vi "GraphsUpdateMeta.vi"(0 "raw graph ref":refnum<vi>, 1 "File Paths":T2={"Local Save Path"=path "\\\\smbhome.uscs.susx.ac.uk\\cv222/Desktop/data", "Newton Save Path"=path "Z:/#Projects/Entanglement/data", "File Name"="test", "LocalSave"=TRUE}, 3 "Compiler Settings":T1={"Python Path"=path "", "Main File"="mainscript.py", "Meta File"="metascript.txt", "Aux File"="auxscript.py", "Pre File"="metascript.txt"}, 5 "mean graph ref":refnum<vi>, 7 "proc graph ref":refnum<vi>, 11 "error in (no error)":errorcluster, 12 "ControllerSettingsRef":refnum<vi>) -> (15 "error out":errorcluster)   [LabVIEW 2019]
uses:
  controls/FilePaths.ctl
  PulseCompiler/CompilerSettings.ctl
  controls/ControllerSettings.ctl
  controls/GlobalExp.vi
  Global.lvlib
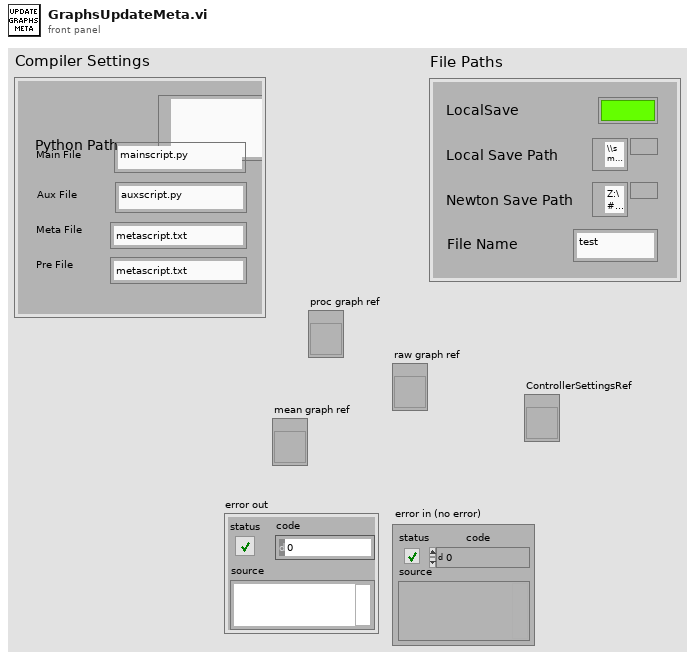
[diagram p1: front panel]
types:
  T1 = typedef "CompilerSettings.ctl" = cluster{"Python Path":path, "Main File":string, "Meta File":string, "Aux File":string, "Pre File":string}
  T2 = typedef "FilePaths.ctl" = cluster{"Local Save Path":path, "Newton Save Path":path, "File Name":string, "LocalSave":bool}
  T3 = typedef "MasterExpControl.ctl" = cluster{"Main Steps":dbl, "Main Runs":dbl, "ExpStatus":enum16{"Innit", "Stop", "Idle", "MainRunning", "AuxRunning"}, "Main Current Step":dbl, "ExpNum":dbl, "NewData":bool, "date":string, "command":string, "Stop":bool, "Pause":bool, "Mathematica":string, "Main/Meta":bool, "UpdateMath":bool, "Camera":bool, "MetaExpOver":bool, "NextMetaExp":bool}
  T4 = typedef "ControllerSettings.ctl" = cluster{"Aux Sequence":bool, "Camera":bool, "Recrystallize":bool, "Raw graph":bool, "Mean graph":bool, "Calculate probs":bool, "Find fit":bool, "ReX Time [s] :":dbl, "Lock Voltage :":dbl, "Line trig ":bool, "Check Fluo":bool, "Pre Sequence":bool}
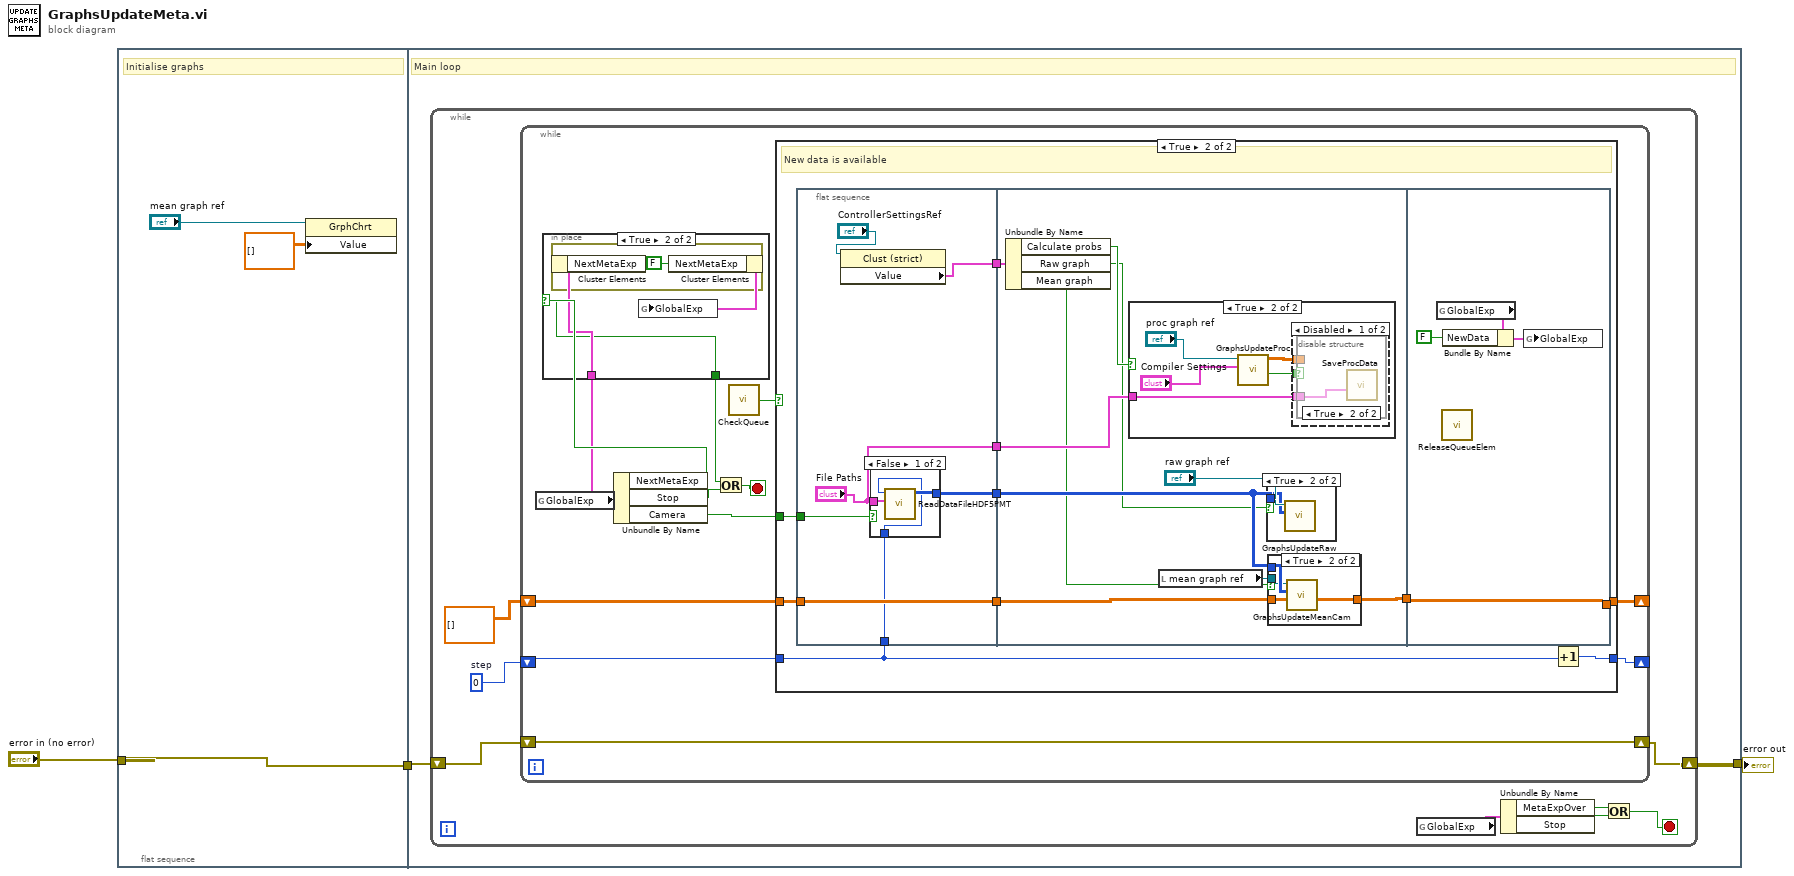
[diagram p0: block diagram]
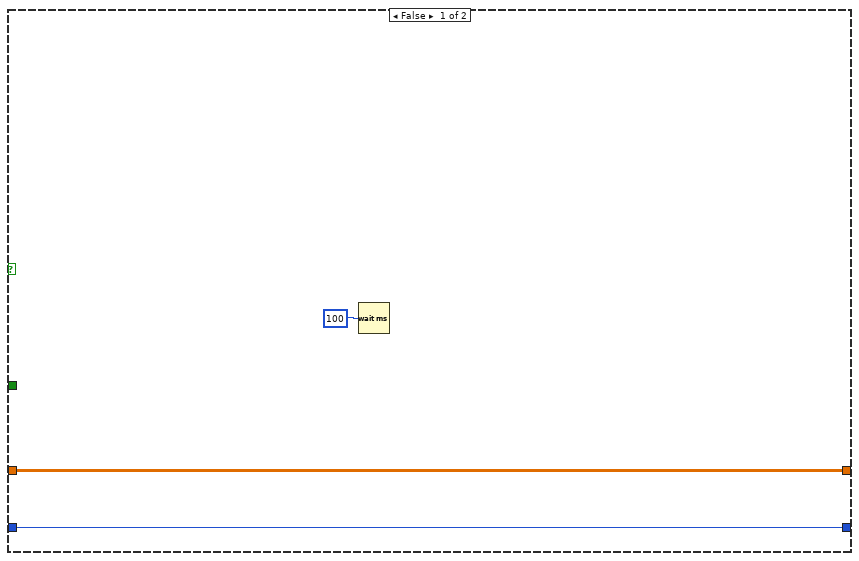
[diagram p3: hidden frame]
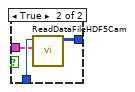
[diagram p4: hidden frame]
diagram:
  n1 = flat-sequence {
    tunnel: "error in (no error)" -> [w6]
    tunnel: [w6] -> w1
    tunnel: [w7] -> w2
    tunnel: w1 -> [w8]
    frame #0 {
      # "Initialise graphs"
      n2 = property class="GrphChrt"(reference="mean graph ref", "Value"=dbl[][] []) -> ()  [unwired: 1 in, 2 out]
    }
    frame #1 {
      # "Main loop"
      n3 = while {
        shift-right: [w15] -> w7
        shift-left: w8 -> [w16]
        stop <- w9 stop-if-true
        w14 = 0  # step
        n4 = while {
          shift-right: [w28] -> w15
          shift-left: w16 -> [w28]
          shift-right: [w24] -> _
          shift-left: w14 -> [w25]
          shift-right: [w22] -> _
          shift-left: dbl[][] [] -> [w23]
          stop <- w17 stop-if-true
          n5 = global read "GlobalExp.vi" "GlobalExp"() -> (w20:T3)
          n6 = Unbundle By Name(w20) -> ("NextMetaExp"=w21:bool, "Stop"=w18:bool, "Camera"=w27:bool)
          n7 = case shown="True" w21 {
            selector: w21 -> [w29 w30]
            tunnel: w20 -> [_ w32]
            tunnel: [w29 w30] -> w19
            frame False {
            }
            frame True {
              n8 = in-place {
                n9 = in-place-cluster #1(w32) -> ()  [unwired: 1 out]
                n10 = in-place-cluster #1("NextMetaExp"=FALSE) -> (w31:T3)
              }
              n11 = global write "GlobalExp.vi" "GlobalExp"(w31) -> ()
            }
          }
          n12 = Or(x=w19, y=w18) -> (x .or. y?=w17:bool)
          n13 = call "CheckQueue.vi"() -> ("x > 0?"=w26:bool)
          n14 = case shown="True" w26 {
            tunnel: w27 -> [_ w38]
            tunnel: w25 -> [w35 w43]
            tunnel: [w35 w46] -> w24
            tunnel: w23 -> [w34 w45]
            tunnel: [w34 w39] -> w22
            frame False {
              n15 = Wait (ms)(milliseconds to wait=u32 100) -> ()  [unwired: 1 out]
            }
            frame True {
              # "New data is available"
              n16 = flat-sequence {
                tunnel: w45 -> [w53]
                tunnel: [w53] -> w44
                tunnel: w43 -> [w52]
                tunnel: [w51] -> w42
                tunnel: ["File Paths"] -> w41
                tunnel: w38 -> [w49]
                tunnel: [w47] -> w37
                tunnel: w44 -> [w69]
                tunnel: w42 -> [w66]
                tunnel: w41 -> [w67]
                tunnel: [w64] -> w40
                tunnel: w37 -> [w62]
                tunnel: w40 -> [w86]
                tunnel: [w86] -> w39
                frame #0 {
                  n17 = property class="Clust (strict)"(reference="ControllerSettingsRef") -> ("Value"=w47:T4)  [unwired: 1 in, 2 out]
                  n18 = case shown="False" w49 {
                    tunnel: w52 -> [w54 w59]
                    tunnel: [w56 w58] -> w51
                    tunnel: "File Paths" -> [w55 w57]
                    frame False {
                      n19 = call "ReadDataFileHDF5PMT.vi"("File Paths"=w55, "step"=w54) -> ("last step data"=w56:i32[][])  [unwired: 8 in, 1 out]
                    }
                    frame True {
                      n20 = call "ReadDataFileHDF5Cam.vi"("File Paths"=w57, "step"=w59) -> ("last step data"=w58:i32[][])  [unwired: 8 in, 1 out]
                    }
                  }
                }
                frame #1 {
                  n21 = Unbundle By Name(w62) -> ("Calculate probs"=w63:bool, "Raw graph"=w61:bool, "Mean graph"=w60:bool)
                  n22 = case shown="True" w63 {
                    tunnel: w67 -> [_ w71]
                    frame False {
                    }
                    frame True {
                      n23 = call "GraphsUpdateProc.vi"("Compiler Settings"="Compiler Settings", "proc graph ref"="proc graph ref") -> ("SaveToCSV?"=w73:bool, "Array"=w74:dbl[][])  [unwired: 8 in]
                      n24 = disable-structure shown="Disabled" {
                        disable-tunnel: w74 -> [w77 _]
                        disable-tunnel: w73 -> [w76 _]
                        disable-tunnel: w71 -> [w75 _]
                        frame Disabled {
                          n25 = case shown="True" w76 {
                            tunnel: w77 -> [_ _]
                            tunnel: w75 -> [_ w78]
                            frame False {
                            }
                            frame True {
                              n26 = call "SaveProcData.vi"("File Paths"=w78) -> ()  [unwired: 11 in]
                            }
                          }
                        }
                        frame Enabled {
                        }
                      }
                    }
                  }
                  n27 = local read "mean graph ref"() -> (w65:refnum<vi>)
                  n28 = case shown="True" w61 {
                    tunnel: "raw graph ref" -> [_ w85]
                    tunnel: w66 -> [_ w84]
                    frame False {
                    }
                    frame True {
                      n29 = call "GraphsUpdateRaw.vi"("data in"=w84, "GraphChart in"=w85) -> ()  [unwired: 10 in]
                    }
                  }
                  n30 = case shown="True" w60 {
                    tunnel: w69 -> [w79 w83]
                    tunnel: w66 -> [_ w82]
                    tunnel: w65 -> [_ w81]
                    tunnel: [w79 w80] -> w64
                    frame False {
                    }
                    frame True {
                      n31 = call "GraphsUpdateMeanCam.vi"("Old mean data in"=w83, "run data in"=w82, "GraphChart in"=w81) -> ("New mean data out"=w80:dbl[][])  [unwired: 8 in]
                    }
                  }
                }
                frame #2 {
                  n32 = global read "GlobalExp.vi" "GlobalExp"() -> (w87:T3)
                  n33 = call "ReleaseQueueElem.vi"() -> ()  [unwired: 12 in]
                  n34 = Bundle By Name(cluster=w87, "NewData"=FALSE) -> (w88:T3)
                  n35 = global write "GlobalExp.vi" "GlobalExp"(w88) -> ()
                }
              }
              n36 = Increment(x=w43) -> (x+1=w46:i32)
            }
          }
        }
        n37 = global read "GlobalExp.vi" "GlobalExp"() -> (w12:T3)
        n38 = Unbundle By Name(w12) -> ("MetaExpOver"=w11:bool, "Stop"=w10:bool)
        n39 = Or(x=w11, y=w10) -> (x .or. y?=w9:bool)
      }
    }
  }
  "error out" <- w2
